vi "moveMotorLaser.vi"(1 "error in (no error)":errorcluster, 2 "Time, ms":dbl, 3 "Refnum in":refnum<k21>) -> (0 "error out":errorcluster)   [LabVIEW 2015]
uses:
  <vilib>/DAQmx/write.llb/DAQmx Write (Digital Bool 1Line 1Point).vi
  <vilib>/DAQmx/miscellaneous.llb/DAQmx Fill In Error Info.vi
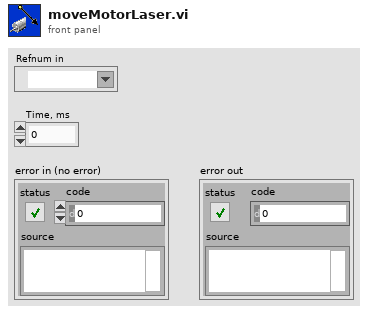
[diagram p1: front panel]
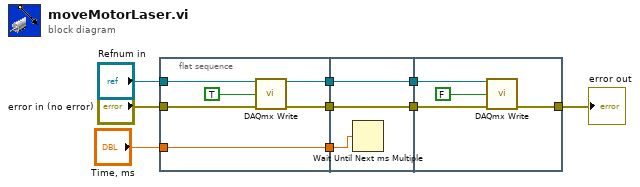
[diagram p0: block diagram]
diagram:
  n1 = flat-sequence {
    tunnel: "Time, ms" -> [w11]
    tunnel: [w14] -> w9
    tunnel: [w13] -> w8
    tunnel: "Refnum in" -> [w12]
    tunnel: [w11] -> w7
    tunnel: "error in (no error)" -> [w10]
    tunnel: w9 -> [w18]
    tunnel: [w18] -> w6
    tunnel: w8 -> [w17]
    tunnel: [w17] -> w5
    tunnel: w7 -> [w16]
    tunnel: w6 -> [w22]
    tunnel: w5 -> [w21]
    tunnel: [w19] -> w3
    frame #0 {
      n2 = call-poly <vilib>:"DAQmx Write.vi"("task/channels in"=w12, "data"=TRUE, "error in"=w10) -> ("task out"=w14:refnum<k21>, "error out"=w13:errorcluster)  [unwired: 10 in, 1 out]
    }
    frame #1 {
      n3 = Wait Until Next ms Multiple(millisecond multiple=w16) -> ()  [unwired: 1 out]
    }
    frame #2 {
      n4 = call-poly <vilib>:"DAQmx Write.vi"("task/channels in"=w22, "data"=FALSE, "error in"=w21) -> ("error out"=w19:errorcluster)  [unwired: 10 in, 2 out]
    }
  }
  "error out" <- w3
